vi "distBetweenPoints.vi"(8 "y2":dbl, 9 "x2":dbl, 10 "y1":dbl, 11 "x1":dbl) -> (2 "d":dbl)   [LabVIEW 2016]
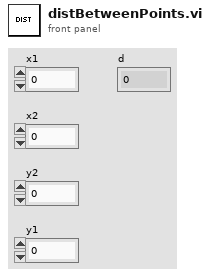
[diagram p1: front panel]
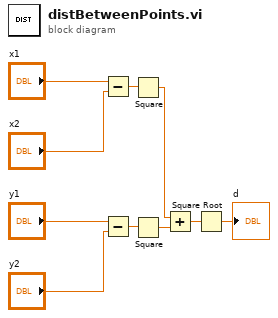
[diagram p0: block diagram]
diagram:
  n1 = Subtract(x="x1", y="x2") -> (x-y=w5:dbl)
  n2 = Subtract(x="y1", y="y2") -> (x-y=w6:dbl)
  n3 = Square(x=w5) -> (x^2=w8:dbl)
  n4 = Square(x=w6) -> (x^2=w7:dbl)
  n5 = Add(x=w8, y=w7) -> (x+y=w9:dbl)
  n6 = Square Root(x=w9) -> (sqrt(x)=→"d":dbl)
